vi "LVIS_Abort.vi"(8 "Error In":errorcluster) -> (0 "Error Out":errorcluster)   [LabVIEW 2015]
doc: "Attempts to close out an incomplete event by setting the Event, Test and Meas Status to Abort. Nothing will be sent if no prior Meas data has been sent or the Event Status is currently not Pending."
uses:
  Sub VIs/Globals/LVIS_IsGlobal.vi
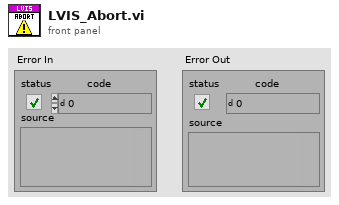
[diagram p1: front panel]
types:
  T1 = cluster{"EventInfo":cluster{"EventName":string, "EventStart":string, "EventStop":string, "EventStatus":string, "EventClientID":string, "IS_EventID":string, "EventMeta":string, "ProductLine":string, "ProcessName":string, "Station":string, "Operator":string, "SN":string, "Model":string, "Manufacturer":string}, "TestInfo":cluster{"TestName":string, "TestDateTime":string, "TestStatus":string, "TestClientID":string, "IS_TestID":string, "TestMeta":string}, "MeasInfo":cluster{"MeasName":string, "MeasDateTime":string, "MeasStatus":string, "MeasClientID":string, "IS_MeasID":string, "MeasMeta":string, "MeasType":string, "MeasValue":string, "LL":string, "LL Comp":string, "HL":string, "HL Comp":string, "Units":string}}[]
  T2 = cluster{"EventInfo":cluster{"EventName":string, "EventStart":string, "EventStop":string, "EventStatus":string, "EventClientID":string, "IS_EventID":string, "EventMeta":string, "ProductLine":string, "ProcessName":string, "Station":string, "Operator":string, "SN":string, "Model":string, "Manufacturer":string}, "TestInfo":cluster{"TestName":string, "TestDateTime":string, "TestStatus":string, "TestClientID":string, "IS_TestID":string, "TestMeta":string}, "MeasInfo":cluster{"MeasName":string, "MeasDateTime":string, "MeasStatus":string, "MeasClientID":string, "IS_MeasID":string, "MeasMeta":string, "MeasType":string, "MeasValue":string, "LL":string, "LL Comp":string, "HL":string, "HL Comp":string, "Units":string}}
  T3 = cluster{"EventName":string, "EventStart":string, "EventStop":string, "EventStatus":string, "EventClientID":string, "IS_EventID":string, "EventMeta":string, "ProductLine":string, "ProcessName":string, "Station":string, "Operator":string, "SN":string, "Model":string, "Manufacturer":string}
  T4 = cluster{"TestName":string, "TestDateTime":string, "TestStatus":string, "TestClientID":string, "IS_TestID":string, "TestMeta":string}
  T5 = cluster{"MeasName":string, "MeasDateTime":string, "MeasStatus":string, "MeasClientID":string, "IS_MeasID":string, "MeasMeta":string, "MeasType":string, "MeasValue":string, "LL":string, "LL Comp":string, "HL":string, "HL Comp":string, "Units":string}
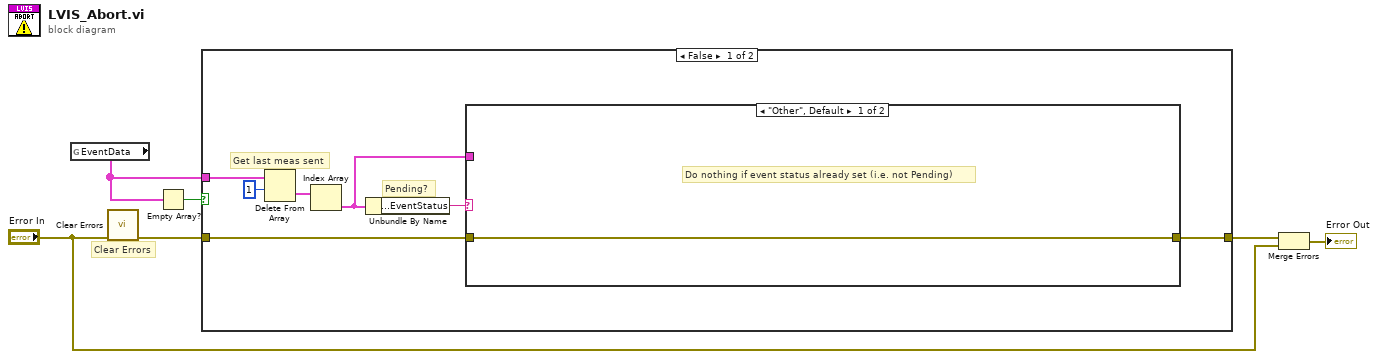
[diagram p0: block diagram]
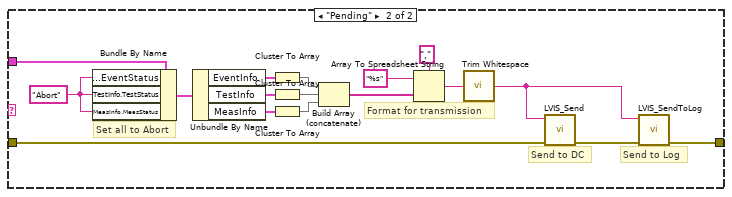
[diagram p2: hidden frame]
diagram:
  # "Clear Errors"
  n1 = global read "LVIS_IsGlobal.vi" "EventData"() -> (w5:T1)
  n2 = call <vilib>:"Clear Errors.vi"("error in (no error)"="Error In") -> ("error out"=w4:errorcluster)  [unwired: 5 in, 1 out]
  n3 = Empty Array?(array=w5) -> (empty?=w6:bool)
  n4 = case shown="False" w6 {
    tunnel: w4 -> [w10 w32]
    tunnel: [w8 w32] -> w3
    tunnel: w5 -> [w13 _]
    frame False {
      # "Pending?"
      # "Get last meas sent"
      n5 = Delete From Array(array=w13, length=1) -> (deleted portion=w11:T1)  [unwired: 1 in, 1 out]
      n6 = Index Array(array=w11) -> (element=w7:T2)  [unwired: 1 in]
      n7 = Unbundle By Name(w7) -> ("EventInfo.EventStatus"=w9:string)
      n8 = case shown="\"Other\", Default" w9 {
        tunnel: w10 -> [w14 w17]
        tunnel: [w14 w15] -> w8
        tunnel: w7 -> [_ w31]
        frame "Other", Default {
          # "Do nothing if event status already set (i.e. not Pending)"
        }
        frame "Pending" {
          w30 = "Abort"
          # "Send to Log"
          # "Send to DC"
          # "Format for transmission"
          # "Set all to Abort"
          n9 = Bundle By Name(cluster=w31, "EventInfo.EventStatus"=w30, "TestInfo.TestStatus"=w30, "MeasInfo.MeasStatus"=w30) -> (w29:T2)
          n10 = Unbundle By Name(w29) -> ("EventInfo"=w28:T3, "TestInfo"=w26:T4, "MeasInfo"=w27:T5)
          n11 = Cluster To Array(cluster=w28) -> (array=w25:string[])
          n12 = Cluster To Array(cluster=w26) -> (array=w24:string[])
          n13 = Cluster To Array(cluster=w27) -> (array=w23:string[])
          n14 = Build Array (concatenate)(w25, w24, w23) -> (w16:string[])
          n15 = Array To Spreadsheet String(delimiter (Tab)=",", array=w16, 3:"%s" ("format string")) -> (spreadsheet string=w20:string)
          n16 = call <vilib>:"Trim Whitespace.vi"("string"=w20) -> ("trimmed string"=w18:string)  [unwired: 1 in]
          n17 = call "LVIS_Send.vi"("Error In"=w17, "Data In"=w18) -> ("Error Out"=w19:errorcluster)  [unwired: 9 in]
          n18 = call "LVIS_SendToLog.vi"("Error In"=w19, "EventData"=w18) -> ("Error Out"=w15:errorcluster)  [unwired: 9 in]
        }
      }
    }
    frame True {
      # "If no data has been sent yet the test has not actually started, so don't send anything"
    }
  }
  n19 = Merge Errors(w3, "Error In") -> (→"Error Out":errorcluster)
